vi "Do Delete Object.vi"(8 "error in (no error)":errorcluster, 10 "delete_object Argument":T2, 11 "Data Cluster in":T1) -> (0 "error out":errorcluster, 3 "Data Cluster out":T1)   [LabVIEW 2025, in "Scripting Server.lvlib"]
uses:
  Scripting Server.lvlib
  delete_object (Reply Payload)--cluster.ctl
  delete_object Argument--cluster.ctl
  Module Data--cluster.ctl
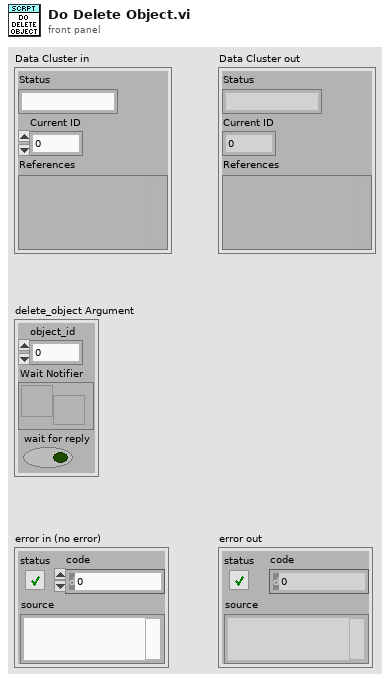
[diagram p1: front panel]
types:
  T1 = typedef "Scripting Server.lvlib/Module Data--cluster.ctl" = cluster{"Status":string, "Current ID":i32, "References":variant}
  T2 = typedef "Scripting Server.lvlib/delete_object Argument--cluster.ctl" = cluster{"object_id":i32, "Wait Notifier":refnum<notifier>, "wait for reply":bool}
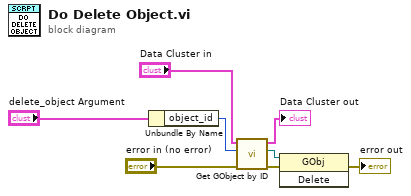
[diagram p0: block diagram]
diagram:
  n1 = Unbundle By Name("delete_object Argument") -> ("object_id"=w3:i32)
  n2 = call "Get GObject by ID.vi"("error in (no error)"="error in (no error)", "ID"=w3, "Data Cluster in"="Data Cluster in") -> ("error out"=w6:errorcluster, "gobject"=w1:refnum<vi>, "Data Cluster out"=→"Data Cluster out":T1)  [unwired: 6 in]
  n3 = invoke class="GObj" method="Delete"(reference=w1, error in=w6) -> (error out=→"error out":errorcluster)  [unwired: 1 in, 2 out]
